vi "Dashboard Main.vi"() -> ()   [LabVIEW 2017]
uses:
  Startpos.ctl
  <vilib>/Utility/miscctls.llb/LVRowAndColumnTypeDef.ctl
  <vilib>/event_ctls.llb/eventvkey.ctl
  <vilib>/Rock Robotics/Network Tables/NT Read Numeric Array.vi
  <vilib>/Rock Robotics/WPI/Dashboard/WPI_DashboardLogging Global.vi
  <vilib>/Rock Robotics/Network Tables/NT Write Boolean.vi
panel:
  in  "Camera Settings Right":T1={"Frame Rate"=30, "Compression"=30, "Size"=1, "DB Camera Config"=FALSE} {"Frame Rate" scale=1.0..30.0; "Compression" scale=100.0..-1.0; "Size" items=["640x480", "320x240", "160x120"]}
  in  "Camera Name Right":string(combo)="No Camera Selection"
  out "Camera Info":cluster{"Mbps LED":bool, "Mbps":dbl, "fps":dbl} {"fps" format="%#.1g"; "Mbps" format="%#.1g"}
  in  "Camera Settings":T1={"Frame Rate"=30, "Compression"=30, "Size"=1, "DB Camera Config"=FALSE} {"Frame Rate" scale=1.0..30.0; "Compression" scale=100.0..-1.0; "Size" items=["640x480", "320x240", "160x120"]}
  in  "TCP":refnum<k5>
  in  "Rec Mode":enum32{"Stop", "Record", "Playback"}(radio)
  out "Robot IP":string
  out "Image Message":string="Timeout in Camera Communications"
  in  "Dashboard Tab":T2(tab)
  in  "Select Auto":string(combo)="Select Autonomous ..."
  out "NT Connection":bool
  out "MotorChart R":cluster{"Numeric":dbl, "Numeric":dbl}(graph)
  out "MotorChart L":cluster{"Numeric":dbl, "Numeric":dbl}(graph)
  out "MotorSliders R":cluster{"MotorSlide1":dbl, "MotorSlide2":dbl} {"MotorSlide2" scale=-1.0..1.0 scale format="%#_2e"; "MotorSlide1" scale=-1.0..1.0 scale format="%#_2e"}
  out "MotorSliders L":cluster{"MotorSlide1":dbl, "MotorSlide2":dbl} {"MotorSlide2" scale=-1.0..1.0 scale format="%#_2e"; "MotorSlide1" scale=-1.0..1.0 scale format="%#_2e"}
  out "Gyro":dbl(knob) scale=0.0..360.0
  out "JS1 Z":dbl(slide) scale=-1.0..1.0 scale format="%#_2e"
  out "JS1 Graph":cluster{"X":dbl, "Y":dbl}[](graph)
  out "JS1 Buttons":T3
  out "JS2 Z":dbl(slide) scale=-1.0..1.0 scale format="%#_2e"
  out "JS2 Graph":cluster{"X":dbl, "Y":dbl}[](graph)
  out "JS2 Buttons":T3
  out "Mode":T4(ring)=enum."Auto Disabled"
  out "Camera Image Right":T5(plugin-control)
  in  "DB/String 9":string
  in  "DB/String 8":string
  in  "DB/String 7":string
  in  "DB/String 6":string
  in  "DB/String 5":string
  in  "DB/String 4":string
  in  "DB/String 3":string
  in  "DB/String 2":string
  in  "DB/String 1":string
  in  "DB/String 0":string
  in  "DB/Slider 0":dbl(slide) scale=0.0..5.0
  in  "DB/Slider 1":dbl(slide) scale=0.0..5.0
  in  "DB/Slider 2":dbl(slide) scale=0.0..5.0
  in  "DB/Slider 3":dbl(slide) scale=0.0..5.0
  out "DB/LED 3":bool
  out "DB/LED 2":bool
  out "DB/LED 1":bool
  out "DB/LED 0":bool
  in  "DB/Button 3":bool
  in  "DB/Button 2":bool
  in  "DB/Button 1":bool
  in  "DB/Button 0":bool caption="New Name"
  out "?":bool
  in  "Start Delay":dbl
  in  "Scale":i32
  in  "Switch":i32
  in  "Alternative placement":bool
  in  "Switch Start":bool
  in  "Scale Start":bool
  in  "Right":bool
  in  "Middle":bool
  in  "Left":bool
  in  "Test Slider":dbl(slide) scale=0.0..100.0 scale format="%#_3g"
  in  "On/Off":bool caption="Solenoid"
  in  "Test Name":u16(ring) items=["Select the test to run..."]
  in  "Test Tree":string(tree)
  in  "Motor":cluster{"Value":dbl, "Enable":bool} {"Value" scale=-1.0..1.0 scale format="%#_3g"}
  out "Progress":T6 {"Test Progress" scale=0.0..100.0}
  in  "Rev/Fwd":cluster{"Forward":bool, "Reverse":bool}
  in  "Test Ring":u16(ring) items=["Monochrome", "Color"]
  out "Cmd Status":string
  in  "Execute Command":bool
  in  "Command Params":string[][](table)
  in  "Command Selection":i32(listbox)
  in  "CheckList":i32(listbox)
  out "Tree":string(tree)
  out "Camera Image":T5(plugin-control)
  out "Background":bool
  in  "Camera Name":string(combo)="No Camera Selection"
  # "HW"
  # "HW"
  # "Joysticks"
  # "Drive Motors"
  # "Front"
  # "Right"
  # "Left"
  # "Back"
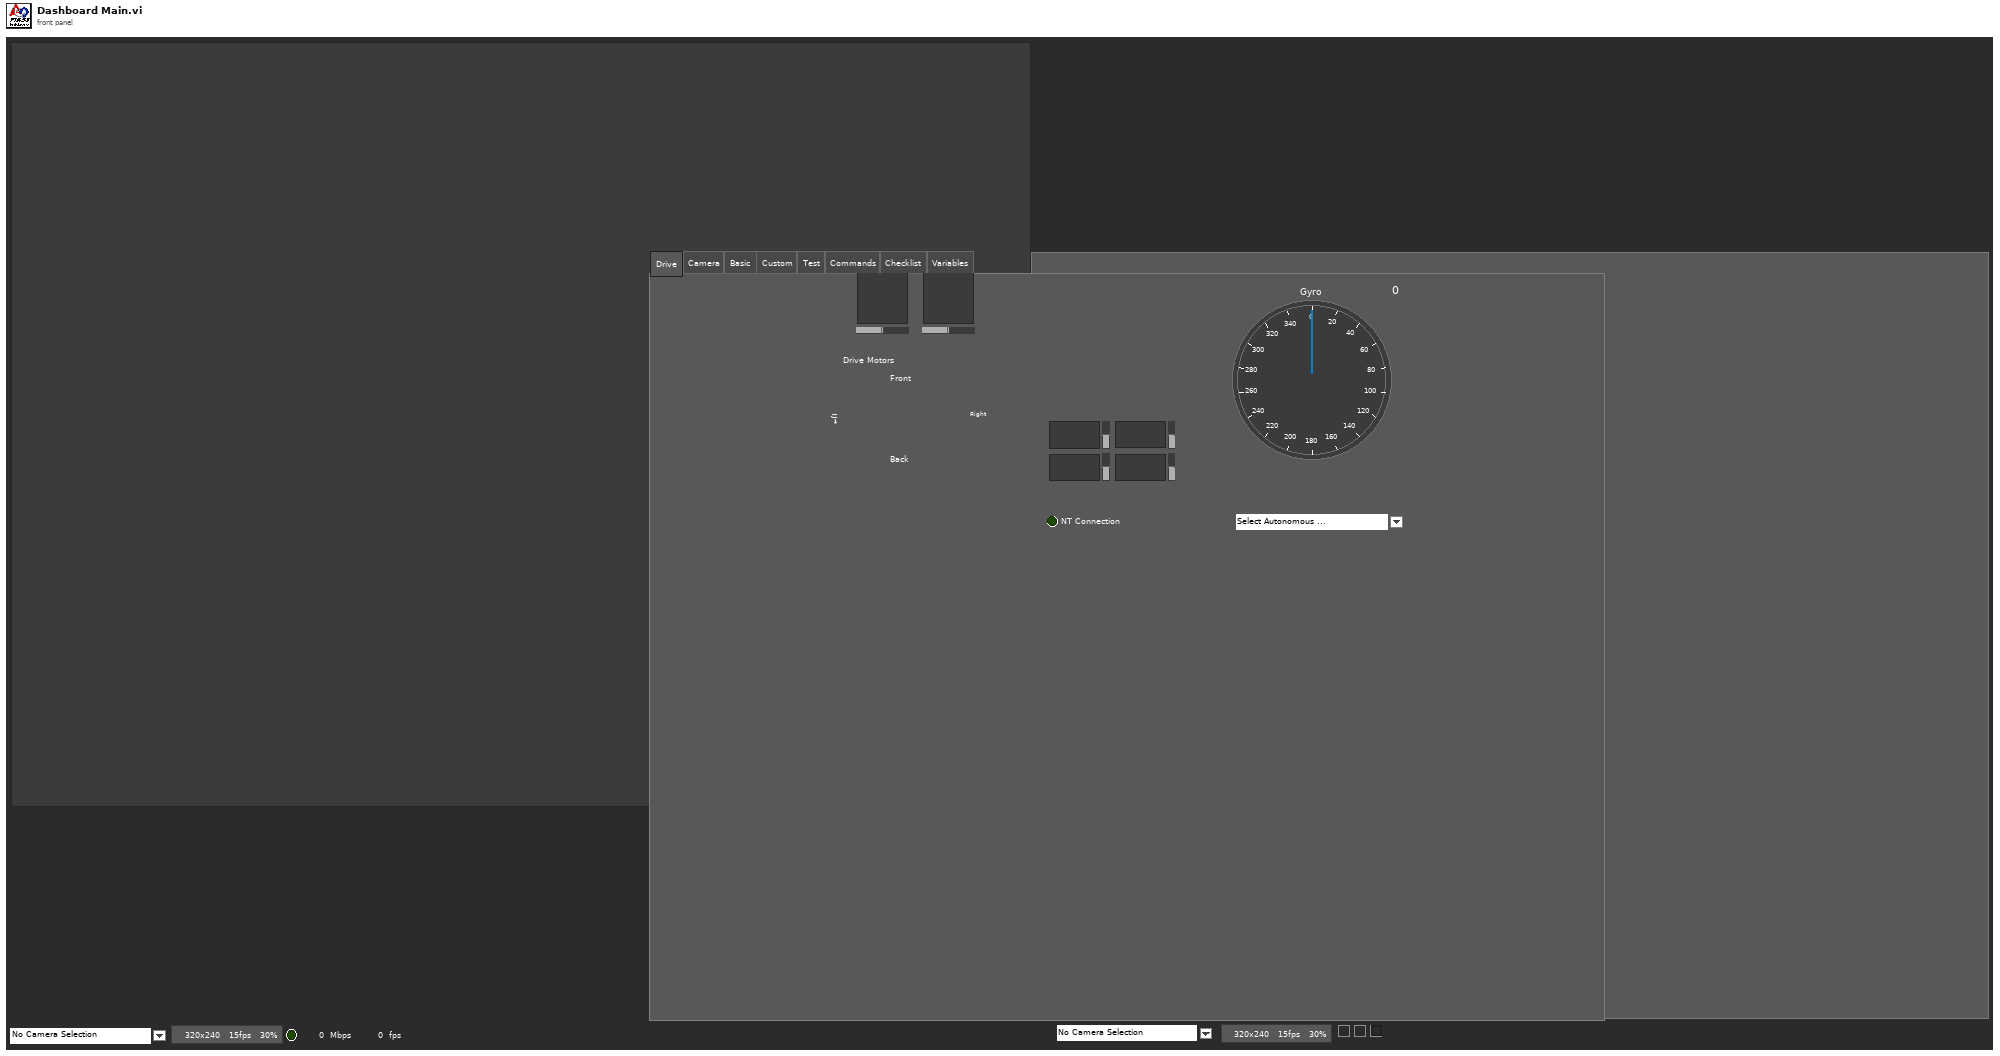
[diagram p1: front panel]
types:
  T1 = cluster{"Frame Rate":i32, "Compression":i32, "Size":u16, "DB Camera Config":bool}
  T2 = enum32{"Drive", "Camera", "Basic", "Custom", "Test", "Commands", "Checklist", "Variables"}
  T3 = cluster{bool, bool, bool, bool, bool, bool, bool, bool, bool, bool, bool, bool}
  T4 = enum8{"Tele-Op Disabled", "Tele-Op Enabled", "Auto Disabled", "Auto Enabled", "Test Disabled", "Test Enabled", "Disconnected", "No Code", "E-Stop"}
  T5 = typedef "IMAQ Image.ctl" = refnum<image>
  T6 = cluster{"Test Progress":u8, "Test Progress Text":string}
  T7 = cluster{"Save Path":path, "Interval (s)":dbl, "Keep":i32}
  T8 = typedef "Image Type" = u32
  T9 = cluster{"IDs":cluster{"RPC field ID":u16, "Unique ID":u16}, "String":string}
  T10 = cluster{"Error Strings":string, "Disable Counts":cluster{u16, u16}, "Rail Faults":cluster{u16, u16, u16}, "Robot IP":string, "DB Mode":u8, "Event Info":cluster{"Name":string, "Type":u8, "Number":u16, "Replay":u8}}
  T11 = cluster{"Storage":cluster{"Disk Free":u64, "RAM Block":u32, "RAM free":u32}, "CPU Utilization":cluster{"CPU % ISR":sgl, "CPU % Time Crit":sgl, "CPU % Timed Str":sgl, "CPU % High":sgl, "CPU % Above":sgl, "CPU % Normal":sgl, "CPU % Low":sgl}, "CAN":cluster{"% Bus Utilization":sgl, "Bus Off Cnt":u32, "TX_FIFO Full Cnt":u32, "Receive Error Cnt":u8, "Transmit Error Cnt":u8}, "HID":cluster{"HID Outputs":u32, "Rumble Low":u16, "Rumble High":u16}[]}
  T12 = cluster{"Status bits":cluster{"Test Mode":bool, "Autonomous":bool, "Enabled":bool, "Code Start":bool, "Brownout":bool, "Reserved 2":bool, "Reserved 3":bool, "E-Stop":bool}, "Code Trace":cluster{"Disabled":bool, "TeleOp":bool, "Auto":bool, "Test":bool}, "Controller Type":enum16{"unknown", "cRIO", "roboRio"}, "Code?":enum16{"unknown", "noCode", "code"}, "Battery V":dbl}
  T13 = cluster{"Control Bits":cluster{"TestMode":bool, "Autonomous":bool, "Enabled":bool, "FMS Present":bool, bool, bool, bool, "E-Stop":bool}, "Team Station ":u8, "Countdown":sgl, "Joystick Values":cluster{"Axes":dbl[], "Buttons":bool[], "POVs":i16[]}[]}
  T14 = cluster{"Axes":dbl[], "Buttons":bool[], "POVs":i16[]}[]
  T15 = cluster{"Axes":dbl[], "Buttons":bool[], "POVs":i16[]}
  T16 = cluster{"Buttons[0]":bool, "Buttons[1]":bool, "Buttons[2]":bool, "Buttons[3]":bool, "Buttons[4]":bool, "Buttons[5]":bool, "Buttons[6]":bool, "Buttons[7]":bool, "Buttons[8]":bool, "Buttons[9]":bool, "Buttons[10]":bool, "Buttons[11]":bool}
  T17 = cluster{"Camera Image":refnum<vi>, "Dashboard Tab":refnum<vi>, "Background":refnum<vi>, "Rec Mode":refnum<vi>, "Test Slider":refnum<vi>, "On/Off ":refnum<vi>, "Test Ring":refnum<vi>, "Rev/Fwd":refnum<vi>, "Test Name":refnum<vi>, "Motor":refnum<vi>, "Progress":refnum<vi>, "CheckList":refnum<vi>, "Tree":refnum<vi>, "Test Tree":refnum<vi>, "Command Params":refnum<vi>, "Command Selection":refnum<vi>, "Execute Command":refnum<vi>, "Cmd Status":refnum<vi>, "Camera Settings":refnum<vi>, "Camera Name":refnum<vi>, "Camera Info":refnum<vi>, "Camera Settings Right":refnum<vi>, "Camera Name Right":refnum<vi>, "Camera Image Right":refnum<vi>}
  T18 = cluster{"Camera Name":string, string, "Saved DB Images Info":cluster{"Save Path":path, "Interval (s)":dbl, "Keep":i32}}
  T19 = cluster{"Camera Name Right":string, string, "Saved DB Images Info":cluster{"Save Path":path, "Interval (s)":dbl, "Keep":i32}}
  T20 = typedef "Startpos.ctl" = enum16{"Left", "Middle", "Right"}
  T21 = cluster{"Operation":enum16{"Update", "Clear"}, "Color Box":u32}[]
  T22 = typedef "eventvkey.ctl" = enum16{"ASCII", "Enter", "Return", "Shift", "Ctrl", "Alt", "Cmd", "Opt", "Caps", "NumLock", "Clear", "Break", "Up", "Down", "Left", "Right", "Insert", "Delete", "Home", "End", "PageUp", "PageDown", "Escape", "Help", "Pause", "ScrollLock", "F1", "F2", "F3", "F4", "F5", "F6", "F7", "F8", "F9", "F10", "F11", "F12", "F13", "F14", "F15", "F16", "F17", "F18", "F19", "F20", "F21", "F22", "F23", "F24", "Play", "VolumeUp", "VolumeDown", "Mute", "Two Byte Char"}
  T23 = cluster{"Image Size":bool, "Image Type":bool, "Pixel Value":bool, "ROI Information":bool, "Zoom Factor":bool}
  T24 = cluster{"Operation":enum16{"Update", "Clear"}, "Color Box":u32}
  T25 = typedef "LVRowAndColumnTypeDef.ctl" = cluster{"Row":i32, "Column":i32}
  T26 = cluster{"Shift":bool, "Ctrl":bool, "Alt":bool, "Cmd":bool, "Opt":bool}
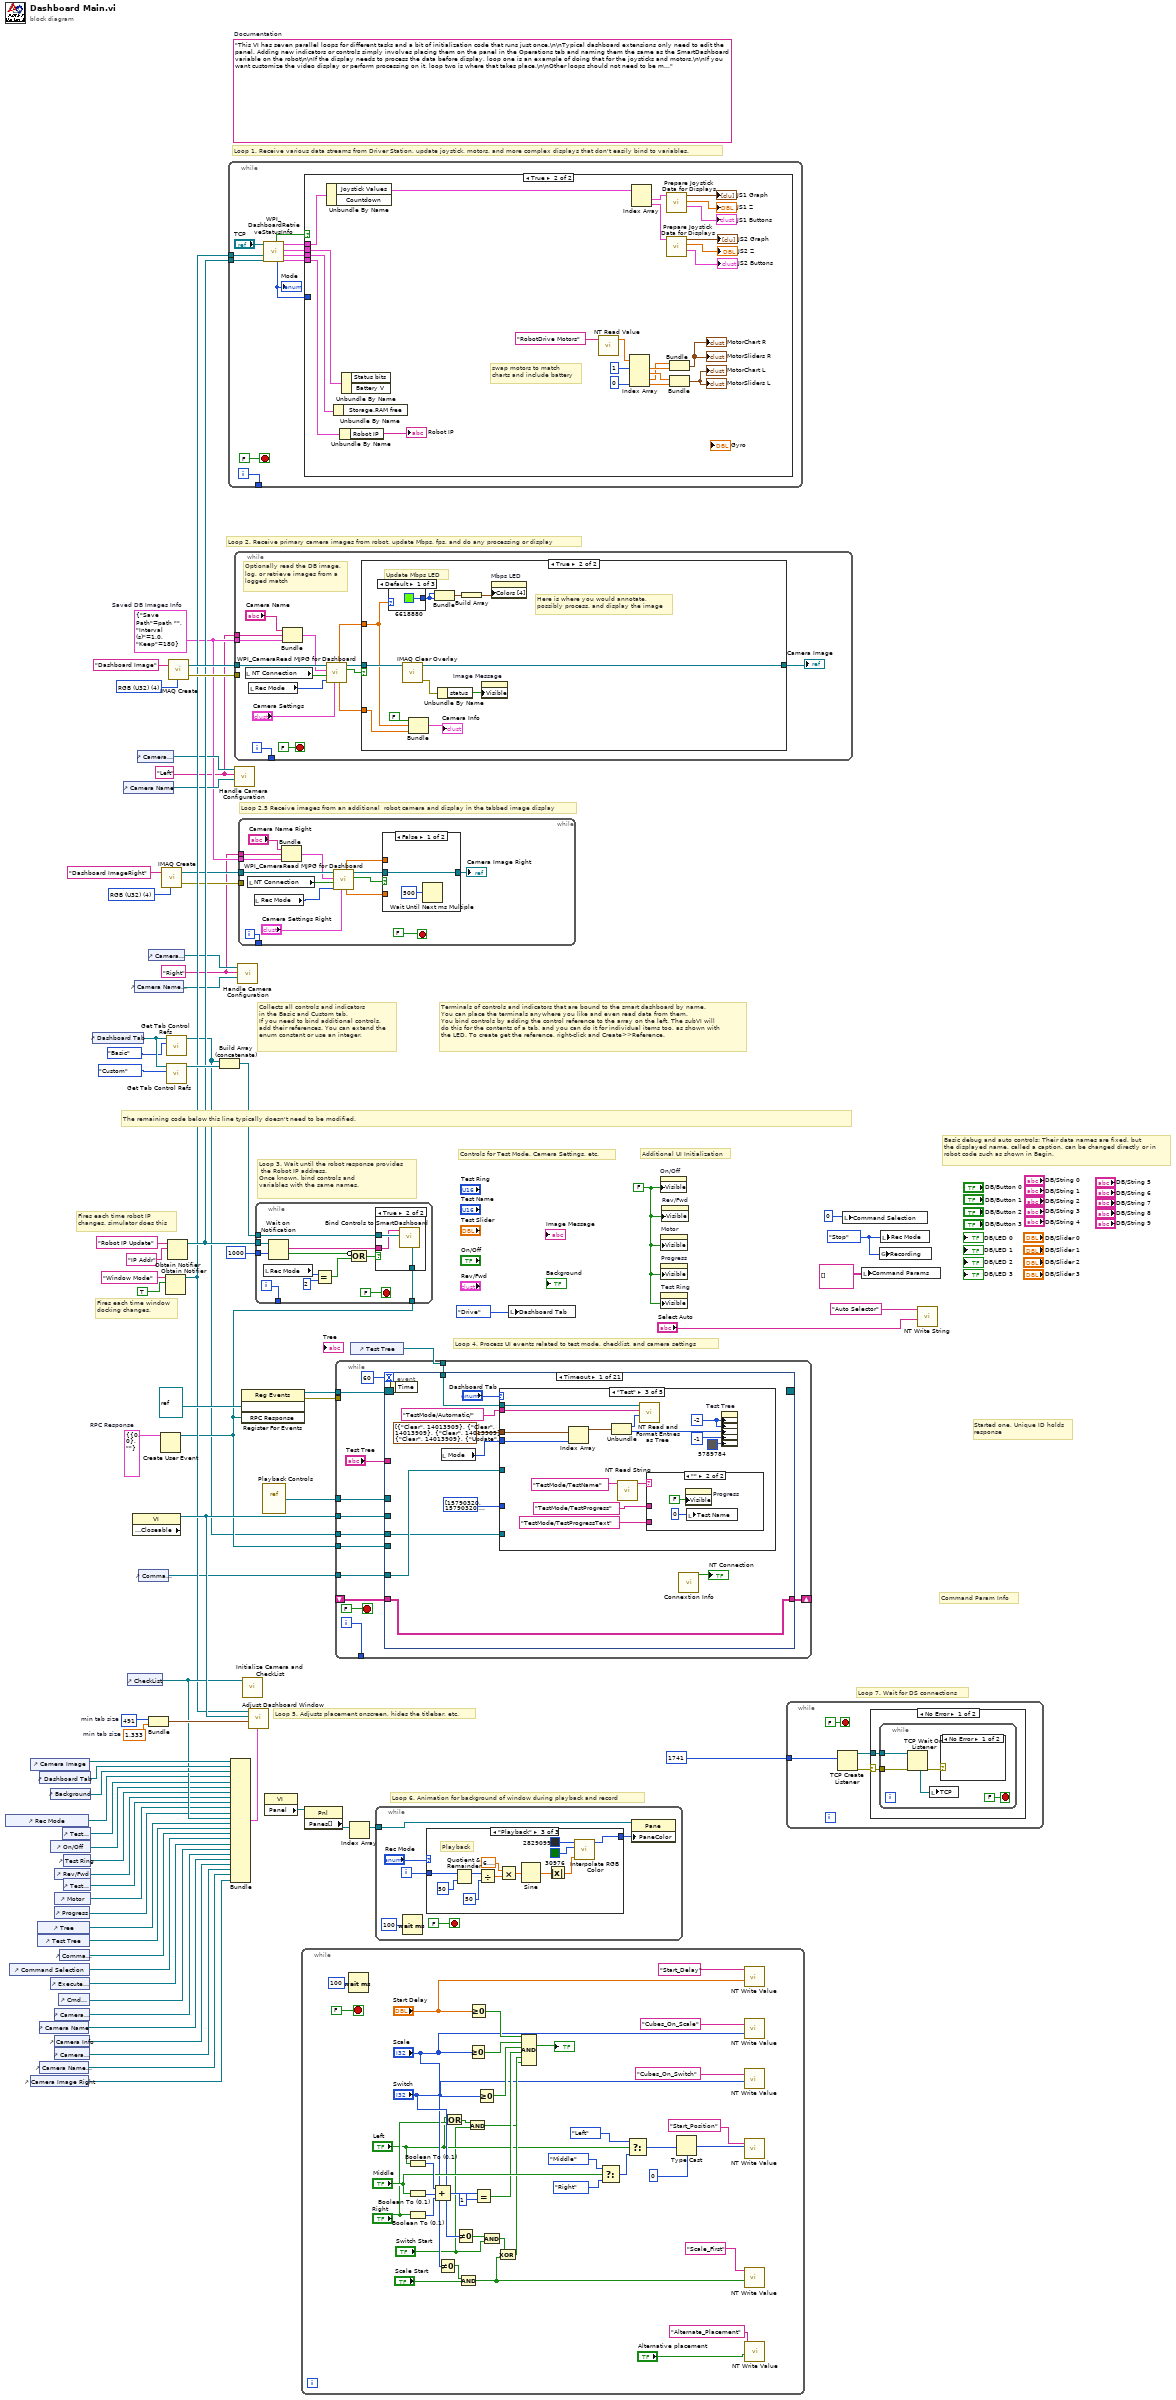
[diagram p0: block diagram]
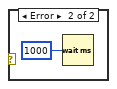
[diagram p3: hidden frame]
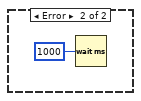
[diagram p4: hidden frame]
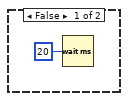
[diagram p5: hidden frame]
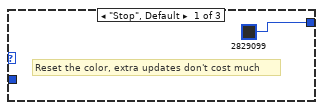
[diagram p6: hidden frame]
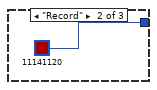
[diagram p7: hidden frame]
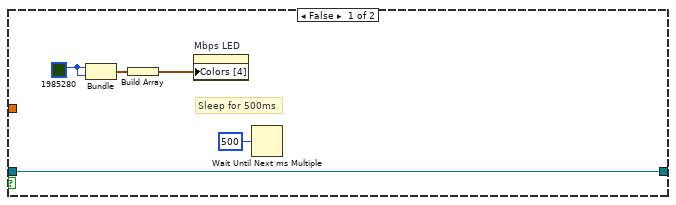
[diagram p9: hidden frame]
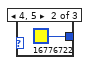
[diagram p10: hidden frame]
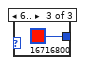
[diagram p11: hidden frame]
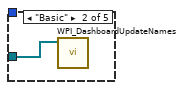
[diagram p13: hidden frame]
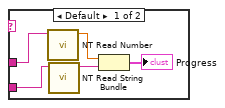
[diagram p14: hidden frame]
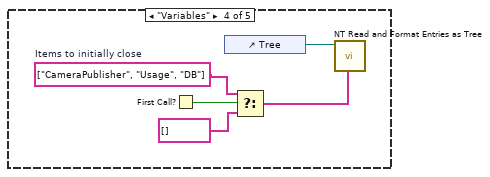
[diagram p15: hidden frame]
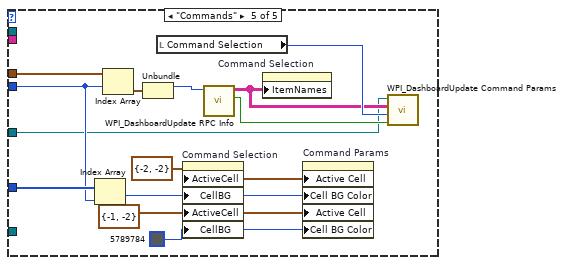
[diagram p16: hidden frame]
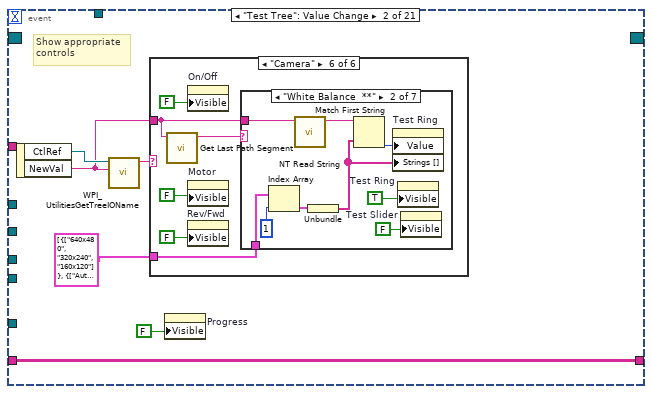
[diagram p17: hidden frame]
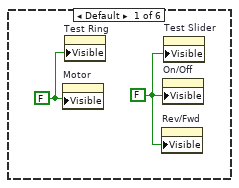
[diagram p18: hidden frame]
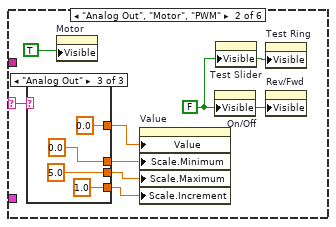
[diagram p19: hidden frame]
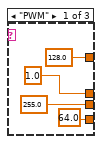
[diagram p20: hidden frame]
diagram:
  w3 = T7 {"Save Path"=path "", "Interval (s)"=1.0, "Keep"=180}  # Saved DB Images Info
  w2 = "Right"
  w1 = "Left"
  w13 = T8 4 items=["Grayscale (U8)", "Grayscale (I16)", "Grayscale (SGL)", "Complex (CSG)", "RGB (U32)", "HSL (U32)", "RGB (U64)"] ("Image Type")
  w29 = T9 {"IDs"={"RPC field ID"=0, "Unique ID"=0}, "String"=""}  # RPC Response
  w52 = 491  # min tab size
  w51 = 1.333  # min tab size
  w59 = enum32{"Stop", "Record", "Playback"}."Stop" ("Rec Mode")
  w36 = FALSE ("Visible")
  (unwired) "This VI has seven parallel loops for different tasks and a bit of initialization code that runs just once.\n\nTypical dashboard extensions only need to edit the panel. Adding new indicators or controls simply involves placing them on the panel in the Operations tab and naming them the same as the SmartDashboard variable on the robot\n\nIf the display needs to process the data before display, loop one is an example of doing that for the joysticks and motors.\n\nIf you want customize the video display or perform processing on it, loop two is where that takes place.\n\nOther loops should not need to be modified. They are pretty standard, and document the task they perform."  # Documentation
  w76 = T8 4 items=["Grayscale (U8)", "Grayscale (I16)", "Grayscale (SGL)", "Complex (CSG)", "RGB (U32)", "HSL (U32)", "RGB (U64)"] ("Image Type")
  # "Loop 2.5 Receive images from an additional  robot camera and display in the tabbed image display"
  # "Command Param Info"
  # "Started one, Unique ID holds\nresponse"
  # "Loop 7. Wait for DS connections"
  # "Basic debug and auto controls: Their data names are fixed, but\nthe displayed name, called a caption, can be changed directly or in\nrobot code such as shown in Begin."
  # "Controls for Test Mode, Camera Settings, etc."
  # "Additional UI Initialization"
  # "Loop 6. Animation for background of window during playback and record"
  # "Fires each time robot IP\nchanges, simulator does this"
  # "Fires each time window\ndocking changes."
  # "Collects all controls and indicators\nin the Basic and Custom tab.\nIf you need to bind additional controls,\nadd their references. You can extend the\nenum constant or use an integer."
  # "The remaining code below this line typically doesn't need to be modified."
  # "Loop 4. Process UI events related to test mode, checklist, and camera settings"
  # "Terminals of controls and indicators that are bound to the smart dashboard by name.\nYou can place the terminals anywhere you like and even read data from them.\nYou bind controls by adding the control reference to the array on the left. The subVI will\ndo this for the contents of a tab, and you can do it for individual items too, as shown with\nthe LED. To create get the reference, right-click and Create>>Reference."
  # "Loop 3. Wait until the robot response provides\n the Robot IP address.\nOnce known, bind controls and\nvariables with the same names."
  # "Loop 5. Adjusts placement onscreen, hides the titlebar, etc."
  # "Loop 1. Receive various data streams from Driver Station, update joystick, motors, and more complex displays that don't easily bind to variables."
  # "Loop 2. Receive primary camera images from robot, update Mbps, fps, and do any processing or display"
  n1 = control-ref of="Rec Mode"() -> (w42:refnum<vi>)
  n2 = control-ref of="Command Selection"() -> (w28:refnum<vi>)
  n3 = control-ref of="Camera Image Right"() -> (w6:refnum<vi>)
  n4 = control-ref of="Camera Image"() -> (w54:refnum<vi>)
  n5 = control-ref of="Tree"() -> (w46:refnum<vi>)
  n6 = control-ref of="Test Tree"() -> (w45:refnum<vi>)
  n7 = control-ref of="Dashboard Tab"() -> (w53:refnum<vi>)
  n8 = control-ref of="Camera Name"() -> (w19:refnum<vi>)
  n9 = control-ref of="Camera Name Right"() -> (w7:refnum<vi>)
  n10 = control-ref of="Execute Command"() -> (w30:refnum<vi>)
  n11 = control-ref of="Background"() -> (w49:refnum<vi>)
  n12 = control-ref of="On/Off"() -> (w40:refnum<vi>)
  n13 = control-ref of="Progress"() -> (w37:refnum<vi>)
  n14 = control-ref of="Camera Settings"() -> (w20:refnum<vi>)
  n15 = control-ref of="Camera Info"() -> (w18:refnum<vi>)
  n16 = control-ref of="Camera Settings Right"() -> (w8:refnum<vi>)
  n17 = control-ref of="Rev/Fwd"() -> (w38:refnum<vi>)
  n18 = control-ref of="Motor"() -> (w43:refnum<vi>)
  n19 = control-ref of="Cmd Status"() -> (w24:refnum<vi>)
  n20 = control-ref of="Command Params"() -> (w31:refnum<vi>)
  n21 = control-ref of="Test Slider"() -> (w41:refnum<vi>)
  n22 = control-ref of="Test Ring"() -> (w39:refnum<vi>)
  n23 = control-ref of="Test Name"() -> (w44:refnum<vi>)
  n24 = control-ref of="Dashboard Tab"() -> (w57:refnum<vi>)
  n25 = control-ref of="Camera Name"() -> (w21:refnum<vi>)
  n26 = control-ref of="CheckList"() -> (w47:refnum<vi>)
  n27 = property class="VI" props=["Front Panel.Closeable"]() -> (reference out=w58:refnum<vi>)  [unwired: 2 in, 2 out]
  n28 = control-ref of="Camera Name Right"() -> (w9:refnum<vi>)
  n29 = control-ref of="Camera Settings"() -> (w22:refnum<vi>)
  n30 = control-ref of="Command Params"() -> (w23:refnum<vi>)
  n31 = control-ref of="Camera Settings Right"() -> (w10:refnum<vi>)
  n32 = Bundle("min tab size"=w52, "min tab size"=w51) -> (w50:cluster{"min tab size":i32, "min tab size":dbl})  [unwired: 1 in]
  n33 = Create User Event(user event datatype=w29) -> (user event=w25:refnum<user-event>)  [unwired: 1 in, 1 out]
  n34 = call "IMAQ Create"("Image Name"="Dashboard ImageRight", "Image Type"=w13) -> ("New Image"=w12:T5, "error out"=w11:errorcluster)  [unwired: 2 in, 1 out]
  n35 = Obtain Notifier(name (unnamed)="Window Mode", notification data type=TRUE) -> (notifier out=w34:refnum<notifier>)  [unwired: 2 in, 2 out]
  n36 = call <vilib>:"Get Tab Control Refs.vi"("Page Index"=T2."Basic" ("Dashboard Tab"), "TabControl in"=w57) -> ("ControlsOnPage"=w17:refnum<vi>[])  [unwired: 9 in]
  n37 = call <vilib>:"Get Tab Control Refs.vi"("Page Index"=T2."Custom" ("Dashboard Tab"), "TabControl in"=w57) -> ("ControlsOnPage"=w56:refnum<vi>[])  [unwired: 9 in]
  n38 = Obtain Notifier(name (unnamed)="Robot IP Update", notification data type="IP Addr" ("name (unnamed)")) -> (notifier out=w35:refnum<notifier>)  [unwired: 2 in, 2 out]
  n39 = call "IMAQ Create"("Image Name"="Dashboard Image", "Image Type"=w76) -> ("New Image"=w74:T5, "error out"=w73:errorcluster)  [unwired: 2 in, 1 out]
  n40 = Build Array (concatenate)(w17, w56) -> (w55:refnum<vi>[])
  n41 = while {
    tunnel: [w86] -> _
    tunnel: w35 -> [w80]
    tunnel: w34 -> [w77]
    i -> [w86]
    stop <- FALSE stop-if-true
    n42 = call <vilib>:"WPI_DashboardRetrieveStatusInfo.vi"("Binding Refnum"=w80, "Window Mode Notifier"=w77, "TCP Cnx"="TCP") -> ("Power and Errors"=w81:T10, "Robot Metrics"=w84:T11, "Status Info"=w85:T12, "Control Info"=w82:T13, "Robot Mode"=w79:T4, "Process?"=w83:bool)  [unwired: 3 in]
    "Mode" <- w79
    n43 = case shown="True" w83 {
      tunnel: w85 -> [_ w112]
      tunnel: w84 -> [_ w111]
      tunnel: w82 -> [_ w110]
      tunnel: w81 -> [_ w109]
      tunnel: w79 -> [_ _]
      frame False {
        n44 = Wait (ms)(milliseconds to wait=u32 20) -> ()  [unwired: 1 out]
      }
      frame True {
        # "swap motors to match\ncharts and include battery"
        n45 = Unbundle By Name(w110) -> ("Joystick Values"=w100:T14)  [unwired: 1 out]
        n46 = Unbundle By Name(w111) -> ()  [unwired: 1 out]
        n47 = Unbundle By Name(w109) -> ("Robot IP"=→"Robot IP":string)
        n48 = Unbundle By Name(w112) -> ()  [unwired: 2 out]
        n49 = call-poly <vilib>:"NT Read Value.vi"("Name"="RobotDrive Motors") -> ("Numeric Array"=w90:dbl[])  [unwired: 9 in, 1 out]
        n50 = Index Array(array=w90, index #1=1, index #4=0) -> (element #1=w104:dbl, element #2=w105:dbl, element #3=w103:dbl, element #4=w108:dbl)  [unwired: 2 in]
        n51 = Index Array(array=w100) -> (element #1=w99:T15, element #2=w95:T15)  [unwired: 2 in]
        n52 = call "Prepare Joystick Data for Displays.vi"("Joystick Values"=w95) -> ("Buttons"=→"JS2 Buttons":T16, "Z Axis"=→"JS2 Z":dbl, "Cartesian Data"=→"JS2 Graph":cluster{"X axis":dbl, "X axis":dbl}[])  [unwired: 8 in]
        n53 = call "Prepare Joystick Data for Displays.vi"("Joystick Values"=w99) -> ("Buttons"=→"JS1 Buttons":T16, "Z Axis"=→"JS1 Z":dbl, "Cartesian Data"=→"JS1 Graph":cluster{"X axis":dbl, "X axis":dbl}[])  [unwired: 8 in]
        n54 = Bundle("Numeric"=w103, "Numeric"=w104) -> (→"MotorChart R" →"MotorSliders R":cluster{"Numeric":dbl, "Numeric":dbl})  [unwired: 1 in]
        n55 = Bundle("Numeric"=w105, "Numeric"=w108) -> (→"MotorChart L" →"MotorSliders L":cluster{"Numeric":dbl, "Numeric":dbl})  [unwired: 1 in]
      }
    }
  }
  n56 = Bundle("Camera Image"=w54, "Dashboard Tab"=w53, "Background"=w49, "Rec Mode"=w42, "Test Slider"=w41, "On/Off"=w40, "Test Ring"=w39, "Rev/Fwd"=w38, "Test Name"=w44, "Motor"=w43, "Progress"=w37, "CheckList"=w47, "Tree"=w46, "Test Tree"=w45, "Command Params"=w31, "Command Selection"=w28, "Execute Command"=w30, "Cmd Status"=w24, "Camera Settings"=w20, "Camera Name"=w19, "Camera Info"=w18, "Camera Settings Right"=w8, "Camera Name Right"=w7, "Camera Image Right"=w6) -> (w48:T17)  [unwired: 1 in]
  n57 = call "Handle Camera Configuration.vi"("CameraNameRef"=w21, "Display Name"=w1, "ClusterRef"=w22) -> ()  [unwired: 9 in]
  n58 = while {
    tunnel: w74 -> [w125]
    tunnel: w73 -> [_]
    tunnel: [w126] -> _
    tunnel: w3 -> [w116]
    tunnel: w1 -> [w113]
    i -> [w126]
    stop <- FALSE stop-if-true
    # "Optionally read the DB image,\nlog, or retrieve images from a\nlogged match"
    n59 = local read "NT Connection"() -> (w117:bool)
    n60 = local read "Rec Mode"() -> (w121:enum32{"Stop", "Record", "Playback"})
    n61 = Bundle("Camera Name"="Camera Name", w113, "Saved DB Images Info"=w116) -> (w115:T18)  [unwired: 1 in]
    n62 = call <vilib>:"WPI_CameraRead MJPG for Dashboard.vi"("Camera Settings"="Camera Settings", "Rec Mode"=w121, "NT Connection"=w117, "Capture Info"=w115, "Refnum in"=w125) -> ("Active"=w123:bool, "Refnum out"=w124:T5, "FPS"=w122:dbl, "Bandwidth (Mbps)"=w120:dbl)  [unwired: 3 in]
    n63 = case shown="True" w123 {
      tunnel: w124 -> [w128 w139]
      tunnel: w120 -> [_ w136]
      tunnel: w122 -> [_ w137]
      tunnel: [w128 w133] -> w118
      frame False {
        w130 = u32 1985280 ("Color Box")
        # "Sleep for 500ms"
        n64 = Bundle("Color Box"=w130, "Color Box"=w130) -> (w131:cluster{"Color Box":u32, "Color Box":u32})  [unwired: 1 out]
        n65 = Build Array(w131) -> (w129:cluster{"Color Box":u32, "Color Box":u32}[])
        n66 = property on="Mbps LED" class="Bool (strict)"("Colors [4]"=w129) -> ()  [unwired: 2 in, 2 out]
        n67 = Wait Until Next ms Multiple(millisecond multiple=u32 500) -> ()  [unwired: 1 out]
      }
      frame True {
        # "Here is where you would annotate,\npossibly process, and display the image"
        # "Update Mbps LED"
        n68 = case shown="Default" w136 {
          tunnel: [u32 6618880 ("Color Box") u32 16776722 ("Color Box") u32 16716800 ("Color Box")] -> w140
          frame Default {
          }
          frame 4, 5 {
          }
          frame 6.. {
          }
        }
        n69 = call "IMAQ Clear Overlay"("Image"=w139) -> ("error out"=w142:errorcluster, "Image Out"=w133:T5)  [unwired: 2 in, 7 out]
        n70 = Bundle(FALSE, "Bandwidth (Mbps)"=w136, "FPS"=w137) -> (→"Camera Info":cluster{bool, "Bandwidth (Mbps)":dbl, "FPS":dbl})  [unwired: 1 in]
        n71 = Bundle("Color Box"=w140, "Color Box"=w140) -> (w141:cluster{"Color Box":u32, "Color Box":u32})  [unwired: 1 out]
        n72 = Unbundle By Name(w142) -> ("status"=w143:bool)
        n73 = Build Array(w141) -> (w138:cluster{"Color Box":u32, "Color Box":u32}[])
        n74 = property on="Image Message" class="Str"("Visible"=w143) -> ()  [unwired: 2 in, 2 out]
        n75 = property on="Mbps LED" class="Bool (strict)"("Colors [4]"=w138) -> ()  [unwired: 2 in, 2 out]
      }
    }
    "Camera Image" <- w118
  }
  n76 = call "Handle Camera Configuration.vi"("CameraNameRef"=w9, "Display Name"=w2, "ClusterRef"=w10) -> ()  [unwired: 9 in]
  n77 = while {
    tunnel: w12 -> [w161]
    tunnel: w11 -> [_]
    tunnel: [w156] -> _
    tunnel: w3 -> [w150]
    tunnel: w2 -> [w147]
    i -> [w156]
    stop <- FALSE stop-if-true
    n78 = local read "NT Connection"() -> (w151:bool)
    n79 = local read "Rec Mode"() -> (w160:enum32{"Stop", "Record", "Playback"})
    n80 = Bundle("Camera Name Right"="Camera Name Right", w147, "Saved DB Images Info"=w150) -> (w149:T19)  [unwired: 1 in]
    n81 = call <vilib>:"WPI_CameraRead MJPG for Dashboard.vi"("Camera Settings"="Camera Settings Right", "Rec Mode"=w160, "NT Connection"=w151, "Capture Info"=w149, "Refnum in"=w161) -> ("Active"=w155:bool, "Refnum out"=w158:T5, "FPS"=w153:dbl, "Bandwidth (Mbps)"=w154:dbl)  [unwired: 3 in]
    n82 = case shown="False" w155 {
      tunnel: w158 -> [w162 w164]
      tunnel: w154 -> [_ _]
      tunnel: w153 -> [_ _]
      tunnel: [w162 w164] -> w152
      frame False {
        n83 = Wait Until Next ms Multiple(millisecond multiple=u32 500) -> ()  [unwired: 1 out]
      }
      frame True {
      }
    }
    "Camera Image Right" <- w152
  }
  n84 = register-events(refnum<vi> refnum, w25) -> (reference out=w63:refnum<event-registration>, error out=w62:errorcluster)  [unwired: 2 in]
  n85 = call "Initialize Camera and CheckList.vi"("ListBox in"=w47) -> ()  [unwired: 11 in]
  n86 = call "Adjust Dashboard Window.vi"("Sizing Refnums"=w48, "Size Constraints"=w50, "VI"=w58, "WIn Mode"=w34) -> ()  [unwired: 8 in]
  n87 = while {
    tunnel: w55 -> [w176]
    tunnel: w35 -> [w174]
    tunnel: [w172] -> _
    tunnel: u32 1000 ("milliseconds to wait") -> [w171]
    tunnel: w25 -> [w165]
    i -> [w172]
    stop <- FALSE stop-if-true
    n88 = local read "Rec Mode"() -> (w167:enum32{"Stop", "Record", "Playback"})
    n89 = Wait on Notification(notifier=w174, timeout in ms (-1)=w171) -> (notification=w173:string, timed out?=w169:bool)  [unwired: 2 in, 2 out]
    n90 = Equal?(x=w167, y=u16 2 ("Rec Mode")) -> (x = y?=w168:bool)
    n91 = Compound Arithmetic op=OR(invert w169, w168) -> (w170:bool)
    n92 = case shown="True" w170 {
      tunnel: w176 -> [_ w179]
      tunnel: w173 -> [_ w178]
      tunnel: w165 -> [_ w177]
      frame False {
      }
      frame True {
        n93 = call <vilib>:"Bind Controls to SmartDashboard.vi"("RPC ref"=w177, "Bound Control Refs"=w179, "Server IP Address"=w178) -> ()  [unwired: 9 in]
      }
    }
  }
  n94 = vi-ref "Playback Controls.vi"() -> (w64:refnum<vi>)
  n95 = property class="VI"() -> ("Panel"=w66:refnum<vi>)  [unwired: 2 in, 2 out]
  n96 = while {
    stop <- FALSE stop-if-true
    n97 = Wait (ms)(milliseconds to wait=u32 100) -> ()  [unwired: 1 out]
    n98 = Boolean To (0,1)(Boolean="Left") -> (0, 1=w197:i16)
    n99 = Boolean To (0,1)(Boolean="Middle") -> (0, 1=w198:i16)
    n100 = Boolean To (0,1)(Boolean="Right") -> (0, 1=w199:i16)
    n101 = Compound Arithmetic op=ADD(w197, w198, w199) -> (w217:i16)
    n102 = Not Equal To 0?(x="Scale") -> (x != 0?=w186:bool)
    n103 = Or(x="Left", y="Right") -> (x .or. y?=w184:bool)
    n104 = Not Equal To 0?(x="Switch") -> (x != 0?=w190:bool)
    n105 = And(x=w186, y="Scale Start") -> (x .and. y?=w188:bool)
    n106 = And(x=w184, y="Switch Start") -> (x .and. y?=w180:bool)
    n107 = Greater Or Equal To 0?(x="Scale") -> (x >= 0?=w219:bool)
    n108 = Greater Or Equal To 0?(x="Start Delay") -> (x >= 0?=w215:bool)
    n109 = Equal?(x=w217, y=i16 1) -> (x = y?=w195:bool)
    n110 = Greater Or Equal To 0?(x="Switch") -> (x >= 0?=w218:bool)
    n111 = And(x=w190, y="Switch Start") -> (x .and. y?=w191:bool)
    n112 = Exclusive Or(1:w188, 2:w191) -> (0:w192:bool)
    n113 = Compound Arithmetic op=AND(w215, w219, w218, w195, w192, w180) -> (→"?":bool)
    n114 = Select(t=Startpos."Middle", s="Middle", f=Startpos."Right") -> (s? t:f=w214:T20)
    n115 = Select(t=Startpos."Left", s="Left", f=w214) -> (s? t:f=w210:T20)
    n116 = Type Cast(type=u16 0, x=w210) -> (*(type *) &x=w203:u16)
    n117 = call-poly <vilib>:"NT Write Value.vi"("Numeric"="Start Delay", "Name"="Start_Delay") -> ()  [unwired: 9 in, 1 out]
    n118 = call-poly <vilib>:"NT Write Value.vi"("Numeric"="Scale", "Name"="Cubes_On_Scale") -> ()  [unwired: 9 in, 1 out]
    n119 = call-poly <vilib>:"NT Write Value.vi"("Numeric"="Switch", "Name"="Cubes_On_Switch") -> ()  [unwired: 9 in, 1 out]
    n120 = call-poly <vilib>:"NT Write Value.vi"("Numeric"=w203, "Name"="Start_Position") -> ()  [unwired: 9 in, 1 out]
    n121 = call-poly <vilib>:"NT Write Value.vi"("Boolean"=w188, "Name"="Scale_First") -> ()  [unwired: 9 in, 1 out]
    n122 = call-poly <vilib>:"NT Write Value.vi"("Boolean"="Alternative placement", "Name"="Alternate_Placement") -> ()  [unwired: 9 in, 1 out]
  }
  n123 = property class="Pnl"(reference=w66) -> ("Panes[]"=w67:refnum<vi>[])  [unwired: 1 in, 2 out]
  n124 = Index Array(array=w67) -> (element=w65:refnum<vi>)  [unwired: 1 in]
  n125 = control-ref of="Test Tree"() -> (w68:refnum<vi>)
  n126 = while {
    tunnel: [w230] -> _
    tunnel: w68 -> [w229]
    tunnel: w64 -> [w228]
    tunnel: w63 -> [w227]
    tunnel: w62 -> [_]
    tunnel: w58 -> [w226]
    tunnel: w25 -> [w225]
    tunnel: w23 -> [w224]
    shift-right: [w223] -> _
    shift-left: _ -> [w222]
    tunnel: w17 -> [w221]
    i -> [w230]
    stop <- FALSE stop-if-true
    n127 = event shown="[0] Timeout" {
      selector: w227 -> [_ _ _ _ _ _ _ _ _ _ _ _ _ _ _ _ _ _ _ _ _]
      dyn-events: [_ _ _ _ _ _ _ _ _ _ _ _ _ _ _ _ w490 _ _ _ _] -> _
      timeout: u32 60 ("milliseconds to wait") -> [_ _ _ _ _ _ _ _ _ _ _ _ _ _ _ _ _ _ _ _ _]
      tunnel: w229 -> [w242 _ _ _ _ _ _ _ _ _ _ _ _ _ _ _ _ _ _ _ _]
      tunnel: "Test Tree" -> [_ _ _ _ _ _ _ _ _ _ _ w457 w465 w467 w471 w479 _ _ _ _ _]
      tunnel: w228 -> [_ _ _ _ _ _ _ _ _ _ _ _ _ _ _ _ w492 _ w510 _ _]
      tunnel: w226 -> [_ _ _ _ _ _ _ _ _ _ _ _ _ _ _ _ w488 _ _ _ _]
      tunnel: w225 -> [_ _ _ _ _ _ _ _ _ _ _ _ _ _ _ _ w486 _ _ _ _]
      tunnel: w224 -> [w237 _ _ _ _ _ w408 _ _ _ _ _ _ _ _ _ _ _ _ _ _]
      tunnel: [w236 w285 w387 w392 w401 w405 w406 w415 w425 w432 w444 w456 w463 w466 w470 w478 w485 w505 w507 w511 w524] -> w223
      tunnel: w222 -> [w236 w285 w387 w392 w401 w405 w406 _ _ w432 w444 w456 w463 w466 w470 w478 w485 w505 w507 w511 w524]
      tunnel: w221 -> [w234 _ _ _ _ _ _ _ _ _ _ _ _ _ _ _ _ _ _ _ _]
      event Timeout {
        n128 = event-data() -> ()  [unwired: 1 in, 1 out]
        n129 = local read "Mode"() -> (w239:T4)
        n130 = case shown="\"Test\"" "Dashboard Tab" {
          tunnel: w242 -> [_ _ w258 _ _]
          tunnel: "TestMode/Automatic/" ("Name Pattern") -> [_ _ w257 _ _]
          tunnel: T21 [{"Operation"=enum."Clear", "Color Box"=14013909}, {"Operation"=enum."Clear", "Color Box"=14013909}, {"Operation"=enum."Clear", "Color Box"=14013909}, {"Operation"=enum."Clear", "Color Box"=14013909}, {"Operation"=enum."Update", "Color Box"=14013909}, {"Operation"=enum."Update", "Color Box"=16777215}, {"Operation"=enum."Clear", "Color Box"=14013909}, {"Operation"=enum."Clear", "Color Box"=14013909}, {"Operation"=enum."Clear", "Color Box"=14013909}] -> [_ _ w250 _ w278]
          tunnel: w239 -> [_ _ w249 _ w277]
          tunnel: u32[] [15790320, 15790320, 15790320, 15790320, 16777215, 16777215, 15790320, 15790320, 15790320] -> [_ _ _ _ w283]
          tunnel: w237 -> [_ _ _ _ w271]
          tunnel: w234 -> [_ w244 _ _ _]
          frame "Custom", Default {
          }
          frame "Basic" {
            n131 = call <vilib>:"WPI_DashboardUpdateNames.vi"("Controls on Tab"=w244) -> ()  [unwired: 11 in]
          }
          frame "Test" {
            w256 = -2 ("Active Item:Row Number")
            n132 = Index Array(array=w250, index=w249) -> (element=w251:T24)
            n133 = Unbundle(w251) -> ("Operation"=w252:enum16{"Update", "Clear"}, "Color Box"=w253:u32)
            n134 = call <vilib>:"NT Read String.vi"("Name"="TestMode/TestName") -> ("String"=w247:string)  [unwired: 9 in, 1 out]
            n135 = call <vilib>:"NT Read and Format Entries as Tree.vi"("Operation"=w252, "Name Pattern"=w257, "Tree Refnum"=w258) -> ()  [unwired: 7 in, 2 out]
            n136 = case shown="\"\"" w247 {
              tunnel: "TestMode/TestProgress" ("Name") -> [w260 _]
              tunnel: "TestMode/TestProgressText" ("Name") -> [w259 _]
              frame Default {
                n137 = call <vilib>:"NT Read Number.vi"("Name"=w260) -> ("Numeric"=w261:dbl)  [unwired: 9 in, 1 out]
                n138 = call <vilib>:"NT Read String.vi"("Name"=w259) -> ("String"=w262:string)  [unwired: 9 in, 1 out]
                n139 = Bundle("Numeric"=w261, "String"=w262) -> (→"Progress":cluster{"Numeric":dbl, "String":string})  [unwired: 1 in]
              }
              frame "" {
                n140 = property on="Progress" class="Clust (strict)"("Visible"=FALSE) -> ()  [unwired: 2 in, 2 out]
                n141 = local write "Test Name"(u16 0) -> ()
              }
            }
            n142 = property on="Test Tree" class="Tree (strict)"("Active Item Row Number"=w256, "ActiveColNum"=w256, "CellBG"=w253, "Active Item Row Number"=-1 ("Active Item:Row Number"), "CellBG"=u32 5789784 ("Color Box")) -> ()  [unwired: 2 in, 2 out]
          }
          frame "Variables" {
            w268 = string[] ["CameraPublisher", "Usage", "DB"]  # Items to initially close
            n143 = First Call?() -> (First Call?: T/F=w269:bool)
            n144 = control-ref of="Tree"() -> (w270:refnum<vi>)
            n145 = Select(t=w268, s=w269, f=string[] []) -> (s? t:f=w266:string[])
            n146 = call <vilib>:"NT Read and Format Entries as Tree.vi"("Tags to  Close"=w266, "Tree Refnum"=w270) -> ()  [unwired: 8 in, 2 out]
          }
          frame "Commands" {
            w279 = u32 5789784 ("Color Box")
            w280 = T25 {"Row"=-1, "Column"=-2} ("Active Cell:Active Cell")
            w282 = T25 {"Row"=-2, "Column"=-2} ("Active Cell:Active Cell")
            n147 = Index Array(array=w283, index=w277) -> (element=w281:u32)
            n148 = Index Array(array=w278, index=w277) -> (element=w276:T24)
            n149 = Unbundle(w276) -> ("Operation"=w275:enum16{"Update", "Clear"})  [unwired: 1 out]
            n150 = local read "Command Selection"() -> (w274:i32)
            n151 = property on="Command Selection" class="MCListbox (strict)"("ActiveCell"=w282, "CellBG"=w281, "ActiveCell"=w280, "CellBG"=w279) -> ()  [unwired: 2 in, 2 out]
            n152 = call <vilib>:"WPI_DashboardUpdate RPC Info.vi"("Operation"=w275) -> ("update"=w273:bool, "commands"=w272:string[][])  [unwired: 9 in]
            n153 = property on="Command Selection" class="MCListbox (strict)"("ItemNames"=w272) -> ()  [unwired: 2 in, 2 out]
            n154 = property on="Command Params" class="Tbl (strict)"("Active Cell"=w282, "Cell BG Color"=w281, "Active Cell"=w280, "Cell BG Color"=w279) -> ()  [unwired: 2 in, 2 out]
            n155 = call <vilib>:"WPI_DashboardUpdate Command Params.vi"("Update"=w273, "NewVal"=w274, "Commands"=w272, "Param Tbl"=w271) -> ()  [unwired: 7 in, 1 out]
          }
        }
        n156 = call <vilib>:"Connextion Info.vi"() -> ("Connected"=→"NT Connection":bool)  [unwired: 10 in, 1 out]
      }
      event "Test Tree": Value Change {
        # "Show appropriate\ncontrols"
        n157 = event-data() -> ("CtlRef"=w288:refnum<vi>, "NewVal"=w286:string)  [unwired: 1 in]
        n158 = call <vilib>:"WPI_UtilitiesGetTreeIOName.vi"("NewVal"=w286, "TreeControl in"=w288) -> ("I/O Name"=w289:string)  [unwired: 9 in]
        n159 = case shown="\"Camera\"" w289 {
          selector: w289 -> [_ w296 _ w318 w327 _]
          tunnel: w286 -> [_ _ w315 w317 _ w334]
          tunnel: cluster{string[]}[] [{["640x480", "320x240", "160x120"]}, {["Auto", "Fixed indoor", "Fixed outdoor 1", "Fixed outdoor 2", "Fixed fluorescent 1", "Fixed fluorescent 2", "Hold current"]}, {["Auto", "Flicker-free 50 Hz", "Flicker-free 60 Hz", "Hold current"]}, {["None", "Prioritize frame rate", "Prioritize image quality"]}, {["Monochrome", "Color"]}] -> [_ _ _ _ _ w333]
          frame Default {
            w291 = FALSE ("Visible")
            w290 = FALSE ("Visible")
            n160 = property on="Motor" class="Clust (strict)"("Visible"=w290) -> ()  [unwired: 2 in, 2 out]
            n161 = property on="Test Ring" class="Ring (strict)"("Visible"=w290) -> ()  [unwired: 2 in, 2 out]
            n162 = property on="Rev/Fwd" class="Clust (strict)"("Visible"=w291) -> ()  [unwired: 2 in, 2 out]
            n163 = property on="On/Off" class="Bool (strict)"("Visible"=w291) -> ()  [unwired: 2 in, 2 out]
            n164 = property on="Test Slider" class="Slide (strict)"("Visible"=w291) -> ()  [unwired: 2 in, 2 out]
          }
          frame "Analog Out", "Motor", "PWM" {
            w297 = FALSE ("Visible")
            n165 = case shown="\"Analog Out\"" w296 {
              tunnel: [1.0 ("Value") -1.0 ("Value") 0.0 ("Value")] -> w295
              tunnel: [255.0 ("Value") 1.0 ("Value") 5.0 ("Value")] -> w294
              tunnel: [128.0 ("Value") 0.0 ("Value") 0.0 ("Value")] -> w293
              tunnel: [64.0 ("Value") 0.5 ("Value") 1.0 ("Value")] -> w292
              frame "PWM" {
              }
              frame "Motor", Default {
              }
              frame "Analog Out" {
              }
            }
            n166 = property on="Motor" class="Clust (strict)"("Visible"=TRUE) -> ()  [unwired: 2 in, 2 out]
            n167 = property on="Value" class="Slide (strict)"("Value"=w293, "Scale.Minimum"=w295, "Scale.Maximum"=w294, "Scale.Increment"=w292) -> ()  [unwired: 2 in, 2 out]
            n168 = property on="On/Off" class="Bool (strict)"("Visible"=w297) -> ()  [unwired: 2 in, 2 out]
            n169 = property on="Test Slider" class="Slide (strict)"("Visible"=w297) -> ()  [unwired: 2 in, 2 out]
            n170 = property on="Test Ring" class="Ring (strict)"("Visible"=w297) -> ()  [unwired: 2 in, 2 out]
            n171 = property on="Rev/Fwd" class="Clust (strict)"("Visible"=w297) -> ()  [unwired: 2 in, 2 out]
          }
          frame "Servo" {
            w313 = FALSE ("Visible")
            n172 = call <vilib>:"NT Read Number.vi"("Name"=w315) -> ("Numeric"=w314:dbl)  [unwired: 9 in, 1 out]
            n173 = property on="Test Slider" class="Slide (strict)"("Visible"=TRUE, "Scale.Maximum"=170.0 ("Scale.Range:Maximum")) -> ()  [unwired: 2 in, 2 out]
            n174 = local write "Test Slider"(w314) -> ()
            n175 = property on="Motor" class="Clust (strict)"("Visible"=w313) -> ()  [unwired: 2 in, 2 out]
            n176 = property on="Rev/Fwd" class="Clust (strict)"("Visible"=w313) -> ()  [unwired: 2 in, 2 out]
            n177 = property on="On/Off" class="Bool (strict)"("Visible"=w313) -> ()  [unwired: 2 in, 2 out]
            n178 = property on="Test Ring" class="Ring (strict)"("Visible"=w313) -> ()  [unwired: 2 in, 2 out]
          }
          frame "Relay", "Solenoid" {
            w316 = FALSE ("Visible")
            n179 = property on="Motor" class="Clust (strict)"("Visible"=w316) -> ()  [unwired: 2 in, 2 out]
            n180 = property on="Test Slider" class="Slide (strict)"("Visible"=w316) -> ()  [unwired: 2 in, 2 out]
            n181 = Search and Replace String(input string=w317, search string="/Value  **", replace string="/Direction") -> (result string=w323:string)  [unwired: 5 in, 3 out]
            n182 = property on="Test Ring" class="Ring (strict)"("Visible"=w316) -> ()  [unwired: 2 in, 2 out]
            n183 = call <vilib>:"NT Read String.vi"("Name"=w323) -> ("String"=w321:string)  [unwired: 9 in, 1 out]
            n184 = Equal?(x="Both directions", y=w321) -> (x = y?=w319:bool)
            n185 = Not(x=w319) -> (.not. x?=w320:bool)
            n186 = property on="Rev/Fwd" class="Clust (strict)"("Visible"=w319) -> ()  [unwired: 2 in, 2 out]
            n187 = property on="On/Off" class="Bool (strict)"("Visible"=w320, "Caption.Text"=w318) -> ()  [unwired: 2 in, 2 out]
          }
          frame "Compressor", "Digital Out" {
            w326 = FALSE ("Visible")
            # "Get direction and finish"
            n188 = property on="Motor" class="Clust (strict)"("Visible"=w326) -> ()  [unwired: 2 in, 2 out]
            n189 = property on="Test Slider" class="Slide (strict)"("Visible"=w326) -> ()  [unwired: 2 in, 2 out]
            n190 = property on="Test Ring" class="Ring (strict)"("Visible"=w326) -> ()  [unwired: 2 in, 2 out]
            n191 = property on="On/Off" class="Bool (strict)"("Visible"=TRUE, "Caption.Text"=w327) -> ()  [unwired: 2 in, 2 out]
            n192 = property on="Rev/Fwd" class="Clust (strict)"("Visible"=FALSE) -> ()  [unwired: 2 in, 2 out]
          }
          frame "Camera" {
            n193 = call <vilib>:"Get Last Path Segment.vi"("String in"=w334) -> ("String out"=w335:string)  [unwired: 10 in]
            n194 = property on="On/Off" class="Bool (strict)"("Visible"=FALSE) -> ()  [unwired: 2 in, 2 out]
            n195 = property on="Motor" class="Clust (strict)"("Visible"=FALSE) -> ()  [unwired: 2 in, 2 out]
            n196 = property on="Rev/Fwd" class="Clust (strict)"("Visible"=FALSE) -> ()  [unwired: 2 in, 2 out]
            n197 = case shown="\"White Balance  **\"" w335 {
              tunnel: w334 -> [w341 w350 w359 w368 w377 _ w383]
              tunnel: w333 -> [w339 w347 w356 w365 w374 _ _]
              frame "Size  **" {
                n198 = Index Array(array=w339) -> (element=w338:cluster{string[]})  [unwired: 1 in]
                n199 = call <vilib>:"NT Read String.vi"("Name"=w341) -> ("String"=w340:string)  [unwired: 9 in, 1 out]
                n200 = Unbundle(w338) -> (w336:string[])
                n201 = Match First String(2:w336, 3:w340) -> (0:w337:i32)  [unwired: 1 out]
                n202 = property on="Test Ring" class="Ring (strict)"("Value"=w337, "Strings []"=w336) -> ()  [unwired: 2 in, 2 out]
                n203 = property on="Test Ring" class="Ring (strict)"("Visible"=TRUE) -> ()  [unwired: 2 in, 2 out]
                n204 = property on="Test Slider" class="Slide (strict)"("Visible"=FALSE) -> ()  [unwired: 2 in, 2 out]
              }
              frame "White Balance  **" {
                n205 = Index Array(array=w347, index=1) -> (element=w348:cluster{string[]})
                n206 = call <vilib>:"NT Read String.vi"("Name"=w350) -> ("String"=w349:string)  [unwired: 9 in, 1 out]
                n207 = Unbundle(w348) -> (w345:string[])
                n208 = Match First String(2:w345, 3:w349) -> (0:w344:i32)  [unwired: 1 out]
                n209 = property on="Test Ring" class="Ring (strict)"("Value"=w344, "Strings []"=w345) -> ()  [unwired: 2 in, 2 out]
                n210 = property on="Test Ring" class="Ring (strict)"("Visible"=TRUE) -> ()  [unwired: 2 in, 2 out]
                n211 = property on="Test Slider" class="Slide (strict)"("Visible"=FALSE) -> ()  [unwired: 2 in, 2 out]
              }
              frame "Exposure  **" {
                n212 = Index Array(array=w356, index=2) -> (element=w357:cluster{string[]})
                n213 = call <vilib>:"NT Read String.vi"("Name"=w359) -> ("String"=w358:string)  [unwired: 9 in, 1 out]
                n214 = Unbundle(w357) -> (w353:string[])
                n215 = Match First String(2:w353, 3:w358) -> (0:w354:i32)  [unwired: 1 out]
                n216 = property on="Test Ring" class="Ring (strict)"("Value"=w354, "Strings []"=w353) -> ()  [unwired: 2 in, 2 out]
                n217 = property on="Test Ring" class="Ring (strict)"("Visible"=TRUE) -> ()  [unwired: 2 in, 2 out]
                n218 = property on="Test Slider" class="Slide (strict)"("Visible"=FALSE) -> ()  [unwired: 2 in, 2 out]
              }
              frame "Exposure Priority  **" {
                n219 = Index Array(array=w365, index=3) -> (element=w366:cluster{string[]})
                n220 = call <vilib>:"NT Read String.vi"("Name"=w368) -> ("String"=w367:string)  [unwired: 9 in, 1 out]
                n221 = Unbundle(w366) -> (w362:string[])
                n222 = Match First String(2:w362, 3:w367) -> (0:w363:i32)  [unwired: 1 out]
                n223 = property on="Test Ring" class="Ring (strict)"("Value"=w363, "Strings []"=w362) -> ()  [unwired: 2 in, 2 out]
                n224 = property on="Test Ring" class="Ring (strict)"("Visible"=TRUE) -> ()  [unwired: 2 in, 2 out]
                n225 = property on="Test Slider" class="Slide (strict)"("Visible"=FALSE) -> ()  [unwired: 2 in, 2 out]
              }
              frame "Color Enable  **" {
                n226 = Index Array(array=w374, index=4) -> (element=w375:cluster{string[]})
                n227 = call <vilib>:"NT Read String.vi"("Name"=w377) -> ("String"=w376:string)  [unwired: 9 in, 1 out]
                n228 = Unbundle(w375) -> (w371:string[])
                n229 = Match First String(2:w371, 3:w376) -> (0:w372:i32)  [unwired: 1 out]
                n230 = property on="Test Ring" class="Ring (strict)"("Value"=w372, "Strings []"=w371) -> ()  [unwired: 2 in, 2 out]
                n231 = property on="Test Ring" class="Ring (strict)"("Visible"=TRUE) -> ()  [unwired: 2 in, 2 out]
                n232 = property on="Test Slider" class="Slide (strict)"("Visible"=FALSE) -> ()  [unwired: 2 in, 2 out]
              }
              frame Default {
                n233 = property on="Test Ring" class="Ring (strict)"("Visible"=FALSE) -> ()  [unwired: 2 in, 2 out]
                n234 = property on="Test Slider" class="Slide (strict)"("Visible"=FALSE) -> ()  [unwired: 2 in, 2 out]
              }
              frame "Brightness  **", "Color Level  **", "Compression  **", "FPS  **", "Sharpness  **" {
                n235 = call <vilib>:"NT Read Number.vi"("Name"=w383) -> ("Numeric"=w382:dbl)  [unwired: 9 in, 1 out]
                n236 = local write "Test Slider"(w382) -> ()
                n237 = property on="Test Slider" class="Slide (strict)"("Visible"=TRUE, "Scale.Maximum"=100.0 ("Scale.Range:Maximum")) -> ()  [unwired: 2 in, 2 out]
                n238 = property on="Test Ring" class="Ring (strict)"("Visible"=FALSE) -> ()  [unwired: 2 in, 2 out]
              }
            }
          }
        }
        n239 = property on="Progress" class="Clust (strict)"("Visible"=FALSE) -> ()  [unwired: 2 in, 2 out]
      }
      event "Test Name": Mouse Enter {
        # "Populate the ring with the list of tests"
        n240 = event-data() -> ()  [unwired: 1 in, 1 out]
        n241 = call <vilib>:"NT Read String Array.vi"("Name"="TestMode/TestList") -> ("String Array"=w391:string[])  [unwired: 9 in, 1 out]
        n242 = Build Array (concatenate)("Select the test to run...", w391) -> (w390:string[])
        n243 = property on="Test Name" class="Ring (strict)"("Strings []"=w390) -> ()  [unwired: 2 in, 2 out]
      }
      event "Test Name": Value Change {
        w393 = FALSE ("Visible")
        # "Tell the robot the test name to run"
        n244 = event-data() -> ("NewVal"=w397:u16)  [unwired: 1 in]
        n245 = property on="Test Name" class="Ring (strict)"() -> ("Strings []"=w398:string[])  [unwired: 2 in, 2 out]
        n246 = local write "Progress"(T6 {"Test Progress"=0, "Test Progress Text"=""} ("Progress")) -> ()
        n247 = Index Array(array=w398, index=w397) -> (element=w396:string)
        n248 = call <vilib>:"NT Write String.vi"("String"=w396, "Name"="TestMode/TestName") -> ()  [unwired: 9 in, 1 out]
        n249 = property on="Progress" class="Clust (strict)"("Visible"=TRUE) -> ()  [unwired: 2 in, 2 out]
        n250 = property on="Motor" class="Clust (strict)"("Visible"=w393) -> ()  [unwired: 2 in, 2 out]
        n251 = property on="Test Slider" class="Slide (strict)"("Visible"=w393) -> ()  [unwired: 2 in, 2 out]
        n252 = property on="On/Off" class="Bool (strict)"("Visible"=w393) -> ()  [unwired: 2 in, 2 out]
        n253 = property on="Rev/Fwd" class="Clust (strict)"("Visible"=w393) -> ()  [unwired: 2 in, 2 out]
        n254 = property on="Test Ring" class="Ring (strict)"("Visible"=w393) -> ()  [unwired: 2 in, 2 out]
      }
      event "Select Auto": Mouse Enter {
        # "Populate the combo box with the list of autonomous options"
        n255 = event-data() -> ()  [unwired: 1 in, 1 out]
        n256 = call <vilib>:"NT Read String Array.vi"("Name"="Auto List") -> ("String Array"=w400:string[])  [unwired: 9 in, 1 out]
        n257 = property on="Select Auto" class="CmbBox"("Strings[]"=w400) -> ()  [unwired: 2 in, 2 out]
      }
      event "Select Auto": Value Change {
        # "User modified the Auto Selection. Write to NT variable so robot knows."
        n258 = event-data() -> ("NewVal"=w403:string)  [unwired: 1 in]
        n259 = call <vilib>:"NT Write String.vi"("String"=w403, "Name"="Auto Selector") -> ()  [unwired: 9 in, 1 out]
      }
      event "Command Selection": Value Change {
        # "Get the params and show in table"
        n260 = event-data() -> ("NewVal"=w409:i32)  [unwired: 1 in]
        n261 = property on="Command Selection" class="MCListbox (strict)"() -> ("ItemNames"=w407:string[][])  [unwired: 2 in, 2 out]
        n262 = call <vilib>:"WPI_DashboardUpdate Command Params.vi"("NewVal"=w409, "Commands"=w407, "Param Tbl"=w408) -> ()  [unwired: 8 in, 1 out]
      }
      event "Execute Command": Value Change {
        # "Started one, Unique ID holds\nresponse"
        n263 = event-data() -> ()  [unwired: 1 in, 1 out]
        n264 = property on="Command Selection" class="MCListbox (strict)"() -> ("ItemNames"=w420:string[][])  [unwired: 2 in, 2 out]
        n265 = Index Array(array=w420, index (row)="Command Selection", index (col)=0) -> (element=w418:string)
        n266 = call <vilib>:"Invoke Commands.vi"("Command Params"="Command Params", "Function Name"=w418) -> ("Params"=w414:u8, "Started"=w413:bool)  [unwired: 7 in, 1 out]
        n267 = Array Subset(array="Command Params", length (row)=w414) -> (w415:string[][])  [unwired: 3 in]
        n268 = Select(t="Executing" ("Cmd Status"), s=w413, f="" ("Cmd Status")) -> (s? t:f=→"Cmd Status":string)
      }
      event "Command Selection": Double Click {
        n269 = event-data() -> ("Row"=w428:i32)  [unwired: 1 in]
        n270 = property on="Command Selection" class="MCListbox (strict)"() -> ("ItemNames"=w431:string[][])  [unwired: 2 in, 2 out]
        n271 = local read "Command Params"() -> (w427:string[][])
        n272 = Index Array(array=w431, index (row)=w428, index (col)=0) -> (element=w429:string)
        n273 = call <vilib>:"Invoke Commands.vi"("Command Params"=w427, "Function Name"=w429) -> ("Params"=w426:u8, "Started"=w421:bool)  [unwired: 7 in, 1 out]
        n274 = Array Subset(array=w427, length (row)=w426) -> (w425:string[][])  [unwired: 3 in]
        n275 = Select(t="Executing" ("Cmd Status"), s=w421, f="" ("Cmd Status")) -> (s? t:f=w422:string)
        n276 = local write "Cmd Status"(w422) -> ()
      }
      event "CheckList": Double Click {
        # "Shift clears all"
        # "Update symbols on the listbox"
        n277 = event-data() -> ("PlatMods.Shift"=w433:bool, "Row"=w435:i32)  [unwired: 1 in]
        n278 = case shown="True" w433 {
          tunnel: w435 -> [w439 _]
          tunnel: 1 -> [w438 _]
          frame False {
            n279 = property on="CheckList" class="LstBox (strict)"() -> ("Item Symbols"=w437:i32[])  [unwired: 2 in, 2 out]
            n280 = Replace Array Subset(array=w437, new element=w438, index=w439) -> (w436:i32[])
            n281 = property on="CheckList" class="LstBox (strict)"("Item Symbols"=w436) -> ()  [unwired: 2 in, 2 out]
          }
          frame True {
            w440 = 0 ("Top Row")
            n282 = property on="CheckList" class="LstBox (strict)"() -> ("Number of Rows"=w442:u32)  [unwired: 2 in, 2 out]
            n283 = Initialize Array(0, w442) -> (w441:i32[])
            n284 = property on="CheckList" class="LstBox (strict)"("Top Row"=w440, "Value"=w440, "Item Symbols"=w441) -> ()  [unwired: 2 in, 2 out]
          }
        }
      }
      event "CheckList": Key Down {
        # "Update symbols on the listbox\nLeft and right keys check and uncheck"
        n285 = event-data() -> ("VKey"=w446:T22)  [unwired: 1 in]
        n286 = case shown="\"Left\", \"Right\"" w446 {
          selector: w446 -> [w451 _]
          tunnel: eventvkey."Left" ("VKey") -> [w449 _]
          frame "Left", "Right" {
            n287 = Equal?(x=w449, y=w451) -> (x = y?=w450:bool)
            n288 = Select(t=0, s=w450, f=1) -> (s? t:f=w452:i32)
            n289 = property on="CheckList" class="LstBox (strict)"() -> ("Item Symbols"=w455:i32[])  [unwired: 2 in, 2 out]
            n290 = Replace Array Subset(array=w455, new element=w452, index="CheckList") -> (w454:i32[])
            n291 = property on="CheckList" class="LstBox (strict)"("Item Symbols"=w454) -> ()  [unwired: 2 in, 2 out]
          }
          frame Default {
          }
        }
      }
      event "Motor.Enable": Value Change {
        # "When the test mode otor enable helper is set, update that\ntree row item's value"
        n292 = event-data() -> ("NewVal"=w461:bool)  [unwired: 1 in]
        n293 = Unbundle("Motor") -> ("Value"=w460:dbl)  [unwired: 1 out]
        n294 = Select(t=w460, s=w461, f=0.0) -> (s? t:f=w458:dbl)
        n295 = call <vilib>:"NT Write Number.vi"("Numeric"=w458, "Name"=w457) -> ()  [unwired: 9 in, 1 out]
      }
      event "Test Slider": Value Change {
        # "When the test mode slider helper is set, update that\ntree row item's value"
        n296 = event-data() -> ("NewVal"=w464:dbl)  [unwired: 1 in]
        n297 = call <vilib>:"NT Write Number.vi"("Numeric"=w464, "Name"=w465) -> ()  [unwired: 9 in, 1 out]
      }
      event "On/Off": Value Change {
        # "When the test mode on/off helper value is set, update that\ntree row item's value"
        n298 = event-data() -> ("NewVal"=w469:bool)  [unwired: 1 in]
        n299 = Boolean To (0,1)(Boolean=w469) -> (0, 1=w468:i16)
        n300 = call <vilib>:"NT Write Number.vi"("Numeric"=w468, "Name"=w467) -> ()  [unwired: 9 in, 1 out]
      }
      event "Rev/Fwd": Value Change {
        # "When the test mode helper value for relays is set, update that\ntree row item's value"
        n301 = event-data() -> ("NewVal.Forward"=w477:bool, "NewVal.Reverse"=w476:bool)  [unwired: 1 in]
        n302 = Boolean To (0,1)(Boolean=w477) -> (0, 1=w473:i16)
        n303 = Boolean To (0,1)(Boolean=w476) -> (0, 1=w475:i16)
        n304 = Negate(x=w475) -> (-x=w474:i16)
        n305 = Add(x=w473, y=w474) -> (x+y=w472:i16)
        n306 = call <vilib>:"NT Write Number.vi"("Numeric"=w472, "Name"=w471) -> ()  [unwired: 9 in, 1 out]
      }
      event "Test Ring": Value Change {
        # "When a test mode helper value is selected from the ring,\nset the tree item's variable to the string value"
        n307 = event-data() -> ("NewVal"=w481:u16)  [unwired: 1 in]
        n308 = property on="Test Ring" class="Ring (strict)"() -> ("Strings []"=w482:string[])  [unwired: 2 in, 2 out]
        n309 = Index Array(array=w482, index=w481) -> (element=w480:string)
        n310 = call <vilib>:"NT Write String.vi"("String"=w480, "Name"=w479) -> ()  [unwired: 9 in, 1 out]
      }
      event "Rec Mode": Value Change {
        # "Update globals for recording mode and path to read log from.\nClear when logging and let NetworkTables set path for vision to\nuse."
        n311 = event-data() -> ("NewVal"=w493:enum32{"Stop", "Record", "Playback"})  [unwired: 1 in]
        n312 = global write "WPI_DashboardLogging Global.vi" "Logging Filename"(path "") -> ()
        n313 = global write "WPI_DashboardLogging Global.vi" "Recording"(w493) -> ()
        n314 = case shown="\"Playback\"" w493 {
          tunnel: w492 -> [_ w495 w504]
          tunnel: [_ _ w503] -> w490
          tunnel: [_ _ w502] -> _
          tunnel: w488 -> [_ _ w500]
          tunnel: cluster{i32, i32} {-250, 170} -> [_ _ w499]
          tunnel: [_ _ T23 {"Image Size"=TRUE, "Image Type"=TRUE, "Pixel Value"=TRUE, "ROI Information"=TRUE, "Zoom Factor"=FALSE} ("Image Information Shown:All Elements")] -> w483
          tunnel: [_ _ TRUE ("Zoom Factor")] -> w484
          tunnel: w486 -> [_ _ w496]
          frame Default {
          }
          frame "Stop", "Record" {
            # "Place Window too"
            n315 = invoke class="VI" method="FP.Close"(reference=w495) -> (reference out=w494:refnum<vi>)  [unwired: 2 in, 2 out]
            n316 = invoke class="VI" method="Abort VI"(reference=w494) -> ()  [unwired: 2 in, 3 out]
          }
          frame "Playback" {
            n317 = call "Open Playback Panel.vi"("Offset"=w499, "DB VI Ref"=w500, "Playback in"=w504) -> ("Playback out"=w501:refnum<vi>)  [unwired: 8 in]
            n318 = register-events(w501, w496) -> (reference out=w503:refnum<event-registration>, error out=w502:errorcluster)  [unwired: 2 in]
          }
        }
        n319 = property on="Camera Image Right" class="ImageControl"("Image Information Shown"=w483, "Image Information Visible"=w484) -> ()  [unwired: 2 in, 2 out]
        n320 = property on="Camera Image" class="ImageControl"("Image Information Shown"=w483, "Image Information Visible"=w484) -> ()  [unwired: 2 in, 2 out]
        n321 = call <vilib>:"WPI_DashboardNT Log FieldName Cache.vi"("Operation"=enum16{"Lookup/Add", "Index", "Clear"}."Clear") -> ()  [unwired: 8 in, 3 out]
      }
      event Panel Close {
        w506 = enum32{"Stop", "Record", "Playback"}."Stop" ("Rec Mode")
        # "Playback window has been closed, abort"
        n322 = event-data() -> ()  [unwired: 1 in, 4 out]
        n323 = local write "Rec Mode"(w506) -> ()
        n324 = global write "WPI_DashboardLogging Global.vi" "Recording"(w506) -> ()
      }
      event Panel Close {
        # "Abort playback window and ourself"
        n325 = event-data() -> ()  [unwired: 1 in, 4 out]
        n326 = invoke class="VI" method="FP.Close"(reference=w510) -> (reference out=w509:refnum<vi>)  [unwired: 2 in, 2 out]
        n327 = invoke class="VI" method="Abort VI"(reference=w509) -> (error out=w508:errorcluster)  [unwired: 2 in, 2 out]
        n328 = invoke class="VI" method="Abort VI"(error in=w508) -> ()  [unwired: 2 in, 3 out]
      }
      event User Event {
        n329 = event-data() -> ("IDs"=w517:cluster{"RPC field ID":u16, "Unique ID":u16}, "String"=w516:string)  [unwired: 1 in]
        n330 = Bundle("IDs"=w517, "String"=w516) -> (w515:T9)  [unwired: 1 in]
        n331 = call <vilib>:"Retrieve RPC Response.vi"("RPC Response"=w515) -> ("Output"=w513:string[][])  [unwired: 10 in]
        n332 = Build Array (concatenate)(w511, w513) -> (w512:string[][])
        n333 = local write "Command Params"(w512) -> ()
        n334 = local write "Cmd Status"("" ("Cmd Status")) -> ()
      }
      event "Tree": Double Click {
        n335 = event-data() -> ("PlatMods"=w523:T26, "Tag"=w520:string)  [unwired: 1 in]
        n336 = Unbundle(w523) -> ("Shift"=w522:bool)  [unwired: 4 out]
        n337 = String Subset(string=w520, length (rest)=1 ("length (rest)")) -> (substring=w519:string)  [unwired: 1 in]
        n338 = Not(x=w522) -> (.not. x?=w521:bool)
        n339 = case shown="\"/\"" w519 {
          tunnel: w520 -> [_ w526]
          tunnel: w521 -> [_ w525]
          frame Default {
          }
          frame "/" {
            n340 = call <vilib>:"NT Update Persistence.vi"("Persistence"=w525, "Name"=w526) -> ()  [unwired: 9 in, 1 out]
          }
        }
      }
    }
  }
  n341 = while {
    tunnel: w65 -> [w528]
    i -> [w531]
    stop <- FALSE stop-if-true
    n342 = Wait (ms)(milliseconds to wait=u32 100) -> ()  [unwired: 1 out]
    n343 = case shown="\"Playback\"" "Rec Mode" {
      tunnel: w531 -> [_ _ w546]
      tunnel: [u32 2829099 ("Base Color") u32 11141120 ("Target Color") w535] -> w527
      frame "Stop", Default {
        # "Reset the color, extra updates don't cost much"
      }
      frame "Record" {
      }
      frame "Playback" {
        # "Playback"
        n344 = Quotient & Remainder(x=w546, y=u32 50 ("milliseconds to wait")) -> (x-y*floor(x/y)=w542:u32)  [unwired: 1 out]
        n345 = Divide(x=w542, y=u32 50 ("milliseconds to wait")) -> (x/y=w539:dbl)
        n346 = Multiply(x=6.283185307179586, y=w539) -> (x*y=w544:dbl)
        n347 = Sine(x=w544) -> (sin(x)=w543:dbl)
        n348 = Absolute Value(x=w543) -> (abs(x)=w536:dbl)
        n349 = call "Interpolate RGB Color.vi"("Proportion"=w536, "Target Color"=u32 30976, "Base Color"=u32 2829099) -> ("Result Color"=w535:u32)  [unwired: 8 in]
      }
    }
    n350 = property class="Pane"(reference=w528, "PaneColor"=w527) -> ()  [unwired: 1 in, 2 out]
  }
  n351 = local write "Dashboard Tab"(T2."Drive" ("Dashboard Tab")) -> ()
  n352 = property on="On/Off" class="Bool (strict)"("Visible"=w36) -> ()  [unwired: 2 in, 2 out]
  n353 = property on="Motor" class="Clust (strict)"("Visible"=w36) -> ()  [unwired: 2 in, 2 out]
  n354 = property on="Progress" class="Clust (strict)"("Visible"=w36) -> ()  [unwired: 2 in, 2 out]
  n355 = property on="Test Ring" class="Ring (strict)"("Visible"=w36) -> ()  [unwired: 2 in, 2 out]
  n356 = property on="Rev/Fwd" class="Clust (strict)"("Visible"=w36) -> ()  [unwired: 2 in, 2 out]
  n357 = while {
    tunnel: u16 1741 ("timeout ms (25000)") -> [w548]
    stop <- FALSE stop-if-true
    n358 = TCP Create Listener(10:w548) -> (0:w547:errorcluster, 3:w549:refnum<k5>)  [unwired: 4 in, 1 out]
    n359 = case shown="No Error" w547 {
      selector: w547 -> [w551 _]
      tunnel: w549 -> [w552 _]
      frame No Error {
        n360 = while {
          tunnel: w552 -> [w555]
          tunnel: w551 -> [w554]
          stop <- FALSE stop-if-true
          n361 = TCP Wait On Listener(8:w554, 11:w555) -> (0:w556:errorcluster, 4:w557:refnum<k5>)  [unwired: 2 in, 3 out]
          n362 = local write "TCP"(w557) -> ()
          n363 = case shown="No Error" w556 {
            frame No Error {
            }
            frame Error {
              n364 = Wait (ms)(milliseconds to wait=u32 1000) -> ()  [unwired: 1 out]
            }
          }
        }
      }
      frame Error {
        n365 = Wait (ms)(milliseconds to wait=u32 1000) -> ()  [unwired: 1 out]
      }
    }
  }
  n366 = local write "Command Selection"(u16 0 ("milliseconds to wait")) -> ()
  n367 = local write "Command Params"(string[][] [] ("Command Params")) -> ()
  n368 = global write "WPI_DashboardLogging Global.vi" "Recording"(w59) -> ()
  n369 = local write "Rec Mode"(w59) -> ()
  n370 = call <vilib>:"NT Write String.vi"("String"="Select Auto", "Name"="Auto Selector") -> ()  [unwired: 9 in, 1 out]
